vi "Async Loop.vi"(1 "RT Data":T1={"Device ref"=0, "Scan Period (uSec)"=10000, "Device Channels"={"Status"={"BD Refs"=[], "Length"=0, "FIFO Index"=0, "Data"=[]}, "Command"={"BD Refs"=[], "Data"=[], "Length"=0, "FIFO Index"=0}}, "Local Chassis"=[], "EtherCAT Masters"=[], "Async"={"Status"=refnum, "Command"=refnum, "Input FIFO"=refnum, "Input FIFO buffer"=[], "Output FIFO"=refnum, "Output FIFO buffer"=[], "Async VI Ref"=refnum}, "ECAT Reconfig"={"Reconfig Module Found"=FALSE, "VI Ref"=refnum, "Status"=refnum}, "Device Error"={"status"=FALSE, "code"=0, "source"=""}, "DeviceName"="", "PCLSync?"=FALSE} {"Device Channels"."Status"."BD Refs"."Data Reference" format="%.0x"; "Device Channels"."Command"."BD Refs"."Data Reference" format="%.0x"; "Local Chassis"."FPGA"."VS ref" format="%.0x"; "Local Chassis"."RSI Modules"."VS ref" format="%.0x"; "Local Chassis"."VS ref" format="%.0x"; "Device ref" format="%.0x"; "EtherCAT Masters"."Generic EtherCAT Slaves"."VS ref" format="%.0x"; "EtherCAT Masters"."VS ref" format="%.0x"; "EtherCAT Masters"."EtherCAT Slaves"."FPGA"."VS ref" format="%.0x"; "EtherCAT Masters"."EtherCAT Slaves"."RSI Modules"."VS ref" format="%.0x"; "EtherCAT Masters"."EtherCAT Slaves"."VS ref" format="%.0x"}) -> ()   [LabVIEW 2016, in "Scan Engine Custom Device.lvlib"]
uses:
  Scan Engine Custom Device.lvlib
  <vilib>/Platform/TimedLoop/XDataNode/XDataNode.xnode
  <vilib>/Platform/TimedLoop/XDataNode/nitl_modes.ctl
  <vilib>/Platform/TimedLoop/XDataNode/XDNodeRunTimeDep.lvlib
  <vilib>/Platform/TimedLoop/XDataNode/wakeup.ctl
  <vilib>/Platform/TimedLoop/XDataNode/timing_clust.ctl
  <vilib>/NI Veristand/Custom Device API/Custom Device API.lvlib
  <vilib>/NI Veristand/Custom Device API/Custom Device Timed Loop Priority.ctl
  Type Defs/Async State.ctl
  Globals/String Constants.vi
  Type Defs/RW Case.ctl
  Type Defs/Async Command.ctl
  <vilib>/Platform/TimedLoop/XDataNode/loadnilvce.vi
  <vilib>/NI Veristand/Custom Device API/Custom Device Item Ref.ctl
  Modules.lvlibp/RSI Module/RSI Module.lvclass
  <vilib>/NI Veristand/Custom Device API/Data Reference.ctl
  <vilib>/NI Veristand/Custom Device API/Block Data Reference.ctl
  Type Defs/Input Data.ctl
  Type Defs/Output Data.ctl
  Modules.lvlibp/RSI Module/Channel Type.ctl
  Type Defs/RSI Module Data.ctl
  Type Defs/FPGA Data.ctl
  Type Defs/Local Chassis Data.ctl
  Type Defs/EtherCAT Slave Data.ctl
  Type Defs/EtherCAT Master Data.ctl
  Type Defs/RT Data.ctl
  Type Defs/Async Status.ctl
  Type Defs/UDV Data Type.ctl
  Type Defs/FXP Config.ctl
  Type Defs/UDV Data.ctl
  Modules.lvlibp/RSI Module/Module Models.ctl
  Type Defs/Module Config Data.ctl
  Type Defs/Async Data.ctl
  Type Defs/ECAT Reconfig State.ctl
  Type Defs/ECAT Reconfig Status.ctl
  Type Defs/ECAT Reconfig Data.ctl
  Type Defs/Device Channels.ctl
  Type Defs/Mixed IO.ctl
  Type Defs/Open Module IOVs.ctl
  Type Defs/Mod Size Indexes.ctl
  Type Defs/Generic ECAT Slave IOV Cluster.ctl
  Type Defs/Generic ECAT Slave Data Cluster.ctl
  Type Defs/Generic ECAT Slave RT-Data-Array.ctl
types:
  T1 = typedef "Scan Engine Custom Device.lvlib/RT Data.ctl" = cluster{"Device ref":T2, "Scan Period (uSec)":u32, "Device Channels":T3, "Local Chassis":T8[], "EtherCAT Masters":T20[], "Async":T25, "ECAT Reconfig":T26, "Device Error":errorcluster, "DeviceName":string, "PCLSync?":bool}
  T2 = typedef "Custom Device API.lvlib/Custom Device Item Ref.ctl" = u64
  T3 = typedef "Scan Engine Custom Device.lvlib/Device Channels.ctl" = cluster{"Status":T4, "Command":T7}
  T4 = typedef "Scan Engine Custom Device.lvlib/Output Data.ctl" = cluster{"BD Refs":T5[], "Length":i32, "FIFO Index":i32, "Data":dbl[]}
  T5 = typedef "Custom Device API.lvlib/Block Data Reference.ctl" = cluster{"Data Reference":T6, "Offset":u64, "Length":u64}
  T6 = typedef "Custom Device API.lvlib/Data Reference.ctl" = i32
  T7 = typedef "Scan Engine Custom Device.lvlib/Input Data.ctl" = cluster{"BD Refs":T5[], "Data":dbl[], "Length":i32, "FIFO Index":i32}
  T8 = typedef "Scan Engine Custom Device.lvlib/Local Chassis Data.ctl" = cluster{"VS ref":T2, "RSI Modules":T9[], "FPGA":T15[], "Input Mod Size Idxs":T19, "Output Modules":i32[], "MixedIO Mod Size Idxs":T19}
  T9 = typedef "Scan Engine Custom Device.lvlib/RSI Module Data.ctl" = cluster{"VS ref":T2, "IOV ref":refnum<k21>, "Open Mod refs":T10, "Module DVR":refnum<data-value>, "Slot":u32, "Model":T11, "Channel Type":T12, "EtherCAT?":bool, "CDInput Data":T7, "CDOutput Data":T4, "Module Config Data":T13, "Mixed IO":T14}
  T10 = typedef "Scan Engine Custom Device.lvlib/Open Module IOVs.ctl" = cluster{"Analog Read":refnum<k21>, "Digital Read":refnum<k21>, "Analog Write":refnum<k21>, "Digital Write":refnum<k21>}
  T11 = typedef "Modules.lvlibp/RSI Module.lvclass/Module Models.ctl" = enum16{"Empty", "NI 9201", "NI 9203", "NI 9205", "NI 9206", "NI 9207", "NI 9208", "NI 9211", "NI 9212", "NI 9213", "NI 9214", "NI 9215", "NI 9217", "NI 9219", "NI 9220", "NI 9221", "NI 9222", "NI 9223", "NI 9225", "NI 9227", "NI 9229", "NI 9233", "NI 9234", "NI 9235", "NI 9236", "NI 9237", "NI 9239", "NI 9242", "NI 9244", "NI 9263", "NI 9264", "NI 9265", "NI 9269", "NI 9375", "NI 9401", "NI 9402", "NI 9403", "NI 9411", "NI 9421", "NI 9422", "NI 9423", "NI 9425", "NI 9426", "NI 9435", "NI 9437", "NI 9472", "NI 9474", "NI 9475", "NI 9476", "NI 9477", "NI 9478", "NI 9481", "NI 9482", "NI 9485"}
  T12 = typedef "Modules.lvlibp/RSI Module.lvclass/Channel Type.ctl" = enum16{"Analog", "Digital"}
  T13 = typedef "Scan Engine Custom Device.lvlib/Module Config Data.ctl" = cluster{"Configurable?":bool, "Config Block Data Refs":T5[], "Config Data DVR":refnum<data-value>, "Previous Values":dbl[], "Local Reconfig VI Ref":refnum<vi>}
  T14 = typedef "Scan Engine Custom Device.lvlib/Mixed IO.ctl" = cluster{"Input Channel Indices":i32[], "Input Buffer":dbl[]}
  T15 = typedef "Scan Engine Custom Device.lvlib/FPGA Data.ctl" = cluster{"VS ref":T2, "IOV ref":refnum<k21>, "FPGA Target":enum16{"Local", "EtherCAT"}, "Product Code":u32, "Bitfile Signature":string, "Bitfile Path (RT)":path, "FPGA Session":u32, "Input Data":T7, "Output Data":T4, "UDVs":cluster{"From FPGA":T16[], "To FPGA":T16[]}}
  T16 = typedef "Scan Engine Custom Device.lvlib/UDV Data.ctl" = cluster{"VS ref":T2, "IOV Ref":refnum<k21>, "Name":string, "UDV Data Type":T17, "Supported Type?":bool, "FXP Config":T18, "FXP VI Ref":refnum<vi>}
  T17 = typedef "Scan Engine Custom Device.lvlib/UDV Data Type.ctl" = enum16{"Boolean", "Fixed Point", "Int8", "Int16", "Int32", "Int64", "U32 Bit Field", "UInt8", "UInt16", "UInt32", "UInt64", "Other"}
  T18 = typedef "Scan Engine Custom Device.lvlib/FXP Config.ctl" = cluster{"signed":bool, "size":u32, "integersize":i32}
  T19 = typedef "Scan Engine Custom Device.lvlib/Mod Size Indexes.ctl" = cluster{"4":i32[], "8":i32[], "16":i32[], "32":i32[], "other":i32[]}
  T20 = typedef "Scan Engine Custom Device.lvlib/EtherCAT Master Data.ctl" = cluster{"VS ref":T2, "IOV ref":refnum<k21>, "Master ID":u32, "Cyclic Data Bandwidth":u32, "EtherCAT Slaves":T21[], "Generic EtherCAT Slaves":T22}
  T21 = typedef "Scan Engine Custom Device.lvlib/EtherCAT Slave Data.ctl" = cluster{"VS ref":T2, "IOV ref":refnum<k21>, "Position Address":u16, "RSI Modules":T9[], "FPGA":T15[], "Input Mod Size Idxs":T19, "Output Modules":i32[], "MixedIO Mod Size Idxs":T19}
  T22 = typedef "Scan Engine Custom Device.lvlib/Generic ECAT Slave RT-Data-Array.ctl" = T23[]
  T23 = typedef "Scan Engine Custom Device.lvlib/Generic ECAT Slave Data Cluster.ctl" = cluster{"VS ref":T2, "IOV ref":refnum<k21>, "Position Address":u16, "I/O Imput Vars ":T24[], "I/O Output Vars":T24[], "I/O Input Data":T7, "I/O Output Data":T4}
  T24 = typedef "Scan Engine Custom Device.lvlib/Generic ECAT Slave IOV Cluster.ctl" = cluster{"VS ref":T2, "IOV Ref":refnum<k21>, "Name":string, "UDV Data Type":T17}
  T25 = typedef "Scan Engine Custom Device.lvlib/Async Data.ctl" = cluster{"Status":refnum<queue>, "Command":refnum<queue>, "Input FIFO":refnum<k33>, "Input FIFO buffer":dbl[], "Output FIFO":refnum<k33>, "Output FIFO buffer":dbl[], "Async VI Ref":refnum<vi>}
  T26 = typedef "Scan Engine Custom Device.lvlib/ECAT Reconfig Data.ctl" = cluster{"Reconfig Module Found":bool, "VI Ref":refnum<vi>, "Status":refnum<queue>}
  T27 = typedef "Scan Engine Custom Device.lvlib/Async State.ctl" = enum16{"Not running", "Waiting on start cmd", "Running", "Paused", "Stopped"}
  T28 = typedef "Scan Engine Custom Device.lvlib/Async Command.ctl" = enum16{"None", "Start", "Stop"}
  T29 = typedef "Custom Device API.lvlib/Custom Device Timed Loop Priority.ctl" = enum32{"Low", "Medium", "High"}
  T30 = typedef "Scan Engine Custom Device.lvlib/RW Case.ctl" = enum16{"Inline read", "Inline write", "Async - Inline loop read", "Async - Inline loop write", "Async loop (read/write)"}
  T31 = typedef "XDNodeRunTimeDep.lvlib/timing_clust.ctl" = cluster{"Expected End [f-1]":u64, "Actual End [f-1]":u64, "Finished Late? [f-1]":bool, "Expected End [i-1]":u64, "Actual End [i-1]":u64, "Finished Late? [i-1]":bool, "Expected Start [i]":u64, "Actual Start [i]":u64, "Expected Start [f]":u64, "Actual Start [f]":u64, "Source Name":string, "Structure Name":string, "Period":i64, "Deadline":i64, "Offset":i64, "Start":i64, "Priority":i32, "Timeout":i32, "Mode":T32, "Wakeup Reason":T33, "Error":errorcluster, "Source Type":string, "Secondary Source Type":string, "Global End Time":u64, "Global Start Time":u64, "Frame Duration":u64, "Iteration Duration":u64, "Assigned CPU":i32, "I/O Scan Engine Mode":u32}
  T32 = typedef "XDNodeRunTimeDep.lvlib/nitl_modes.ctl" = enum32{"No Change", "Process missed periods, maintain original phase", "Discard missed periods, maintain original phase", "Process missed periods, ignore original phase", "Discard missed periods, ignore original phase"}
  T33 = typedef "XDNodeRunTimeDep.lvlib/wakeup.ctl" = enum32{"Normal", "Aborted", "Asynchronous wakeup", "Timing source error", "Timed loop error", "Timeout"}
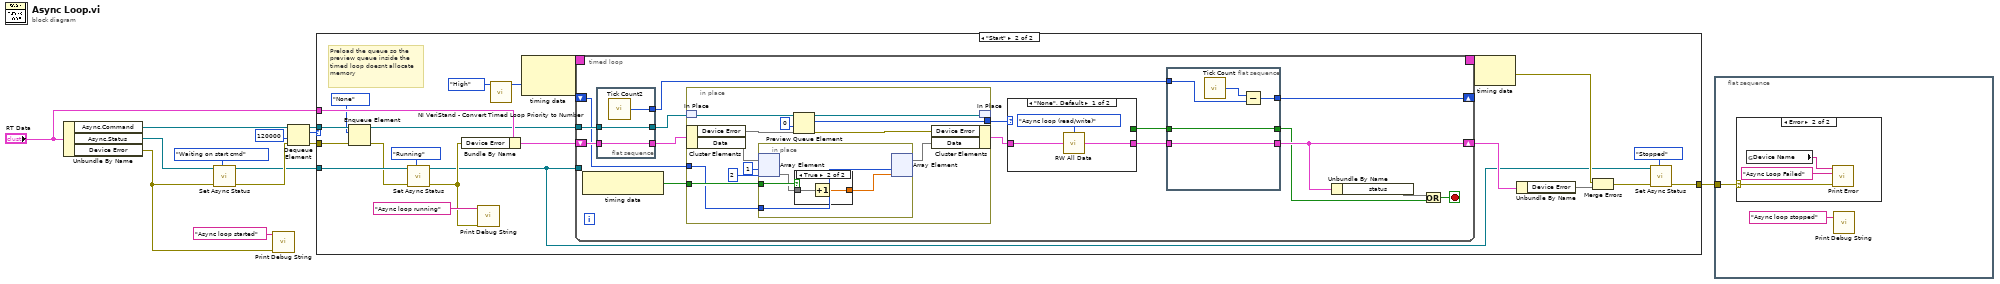
[diagram p0: block diagram]
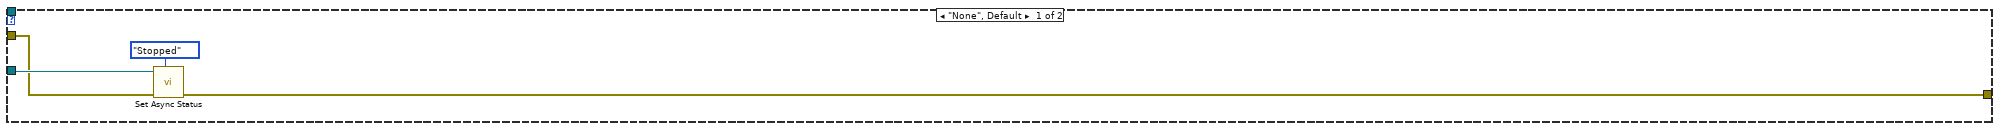
[diagram p3: hidden frame]
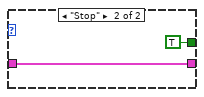
[diagram p4: hidden frame]
diagram:
  n1 = Unbundle By Name("RT Data") -> ("Async.Command"=w8:refnum<queue>, "Async.Status"=w10:refnum<queue>, "Device Error"=w1:errorcluster)
  n2 = call "Set Async Status.vi"("State"=Async_State."Waiting on start cmd", "error in (no error)"=w1, "Status in"=w10) -> ("error out"=w7:errorcluster, "Status out"=w5:refnum<queue>)  [unwired: 7 in]
  n3 = call "Print Debug String.vi"("error in"=w1, "String to write"="Async loop started") -> ()  [unwired: 8 in, 1 out]
  n4 = Dequeue Element(queue=w8, timeout in ms (-1)=120000, error in (no error)=w7) -> (queue out=w6:refnum<queue>, element=w11:T28, error out=w4:errorcluster)  [unwired: 1 out]
  n5 = case shown="\"Start\"" w11 {
    tunnel: "RT Data" -> [_ w33]
    tunnel: w6 -> [_ w20]
    tunnel: w5 -> [w16 w35]
    tunnel: w4 -> [w15 w34]
    tunnel: [w14 w29] -> w3
    frame "None", Default {
      n6 = call "Set Async Status.vi"("State"=Async_State."Stopped", "error in (no error)"=w15, "Status in"=w16) -> ("error out"=w14:errorcluster)  [unwired: 7 in, 1 out]
    }
    frame "Start" {
      # "Preload the queue so the preview queue inside the timed loop doesnt allocate memory"
      n7 = Enqueue Element(queue=w20, element=Async_Command."None", error in (no error)=w34) -> (queue out=w19:refnum<queue>, error out=w21:errorcluster)  [unwired: 1 in, 1 out]
      n8 = call "Set Async Status.vi"("State"=Async_State."Running", "error in (no error)"=w21, "Status in"=w35) -> ("error out"=w24:errorcluster, "Status out"=w22:refnum<queue>)  [unwired: 7 in]
      n9 = Bundle By Name(cluster=w33, "Device Error"=w24) -> (w32:T1)
      n10 = call "Print Debug String.vi"("error in"=w24, "String to write"="Async loop running") -> ()  [unwired: 8 in, 1 out]
      n11 = call <vilib>:"NI VeriStand - Convert Timed Loop Priority to Number.vi"("Priority"=Custom_Device_Timed_Loop_Priority."High") -> ("Numeric Priority"=w36:i32)  [unwired: 10 in]
      n12 = node-c288(w36) -> (w39:T31)  [unwired: 1 in]
      n13 = timed-loop {
        timing: w39 -> [_]
        timing-out: [_] -> w38
        shift-right: [w50] -> w30
        shift-left: w32 -> [w44]
        tunnel: w19 -> [w46]
        tunnel: w22 -> [_]
        shift-right: [w53] -> _
        shift-left: _ -> [w41]
        stop <- w54 stop-if-true
        n14 = node-c288() -> (w42:bool)  [unwired: 1 in]
        n15 = flat-sequence {
          tunnel: w46 -> [w58]
          tunnel: [w58] -> w40
          tunnel: [w57] -> w45
          tunnel: w44 -> [w57]
          tunnel: [w56] -> w43
          frame #0 {
            n16 = call "Tick Count2"() -> ("Tick Count(uSec)"=w56:u32)
          }
        }
        n17 = in-place {
          in-place-border: [w77] -> w51
          in-place-border: w42 -> [w73]
          in-place-border: w41 -> [w72]
          n18 = in-place-match #1(w40) -> (w70:refnum<queue>)
          n19 = in-place-cluster #2(w45) -> ("Device Error"=w79, "Data"=w76)
          n20 = in-place {
            in-place-border: w73 -> [w84]
            in-place-border: w72 -> [w81]
            n21 = in-place-array #3(w76, 1, 2) -> (w83)  [unwired: 1 out]
            n22 = case shown="True" w84 {
              tunnel: w83 -> [w85 w87]
              tunnel: [w85 w86] -> w82
              frame False {
              }
              frame True {
                n23 = Increment(x=w87) -> (x+1=w86:dbl)
              }
            }
            n24 = in-place-array #3(w81, w82) -> (w71)  [unwired: 2 out]
          }
          n25 = Preview Queue Element(queue=w70, timeout in ms (-1)=0, error in (no error)=w79) -> (queue out=w69:refnum<queue>, element=w77:T28, error out=w78:errorcluster)  [unwired: 1 out]
          n26 = in-place-cluster #2("Device Error"=w78, "Data"=w71) -> (w52:cluster{})
          n27 = in-place-match #1(w69) -> ()  [unwired: 1 out]
        }
        n28 = case shown="\"None\", Default" w51 {
          tunnel: [_ TRUE] -> w47
          tunnel: w52 -> [w66 w67]
          tunnel: [w64 w67] -> w49
          frame "None", Default {
            n29 = call "RW All Data.vi"("R/W Case"=RW_Case."Async loop (read/write)", "RT Data in"=w66) -> ("RT Data out"=w64:T1)  [unwired: 13 in]
          }
          frame "Stop" {
          }
        }
        n30 = flat-sequence {
          tunnel: [w63] -> w53
          tunnel: w43 -> [w62]
          tunnel: [w60] -> w50
          tunnel: w49 -> [w60]
          tunnel: [w59] -> w48
          tunnel: w47 -> [w59]
          frame #0 {
            n31 = call "Tick Count"() -> ("Tick Count(uSec)"=w61:u32)
            n32 = Subtract(x=w61, y=w62) -> (x-y=w63:u32)
          }
        }
        n33 = Unbundle By Name(w50) -> ("status"=w55)
        n34 = Or(x=w55, y=w48) -> (x .or. y?=w54:bool)
      }
      n35 = node-c288(w38) -> (w28:errorcluster)
      n36 = Unbundle By Name(w30) -> ("Device Error"=w27)
      n37 = Merge Errors(w28, w27) -> (w26:errorcluster)
      n38 = call "Set Async Status.vi"("State"=Async_State."Stopped", "error in (no error)"=w26, "Status in"=w22) -> ("error out"=w29:errorcluster)  [unwired: 7 in, 1 out]
    }
  }
  n39 = flat-sequence {
    tunnel: w3 -> [w96]
    frame #0 {
      n40 = case shown="Error" w96 {
        selector: w96 -> [_ w98]
        frame No Error {
        }
        frame Error {
          n41 = global read "String Constants.vi" "Device Name"() -> (w100:string)
          n42 = call "Print Error.vi"("error in (no error)"=w98, "Note (empty)"="Async Loop Failed", "Your code's public name"=w100) -> ()  [unwired: 7 in, 1 out]
        }
      }
      n43 = call "Print Debug String.vi"("String to write"="Async loop stopped") -> ()  [unwired: 9 in, 1 out]
    }
  }
